vi "Lines LoadMatrixOfSessions.vi"(8 "error in (no error)":errorcluster, 9 "Input Dialog":string, 10 "Array in":string[](array[string]), 11 "Lines":string[](array[string])) -> (0 "error out":errorcluster, 2 "Array out":string[][](array[string]), 3 "Config Text List out":string[](array[string]))   [LabVIEW 2012]
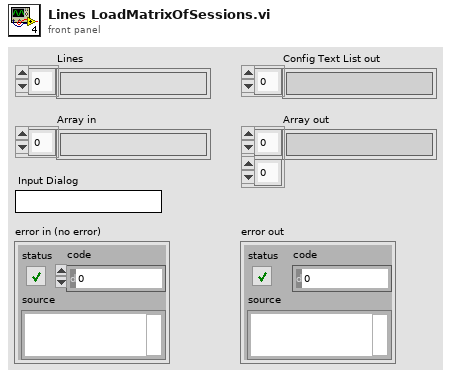
[diagram p1: front panel]
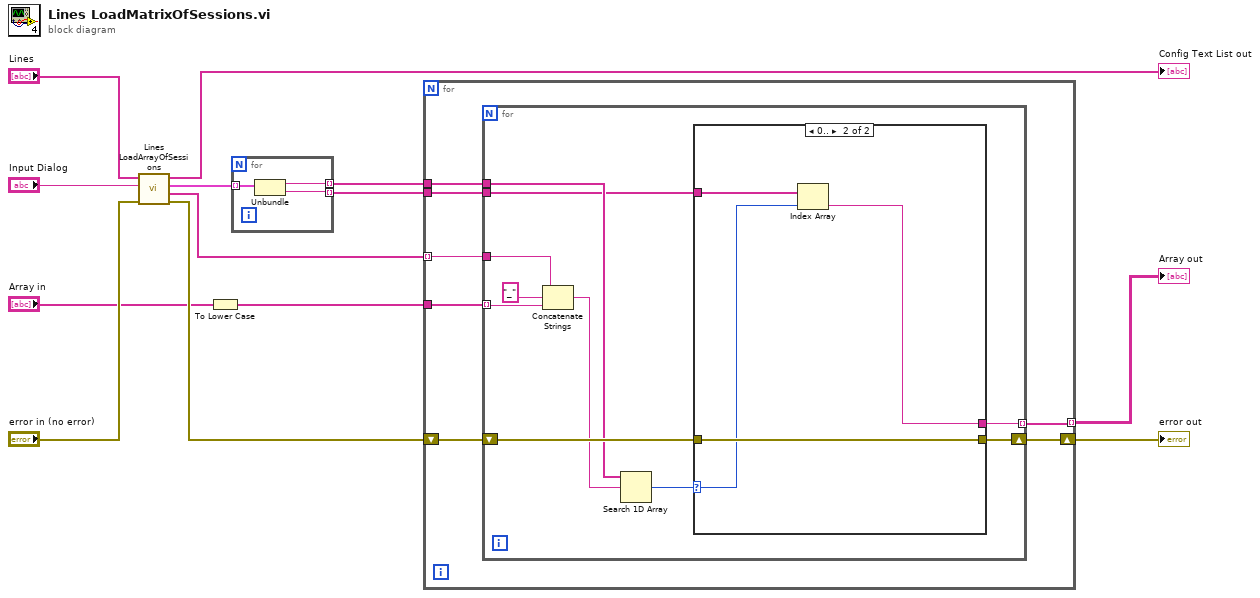
[diagram p0: block diagram]
diagram:
  n1 = call "Lines LoadArrayOfSessions.vi"("error in (no error)"="error in (no error)", "regular expression"="Input Dialog", "Lines"="Lines") -> ("error out"=w11:errorcluster, "Matched Sessions"=w6:string[], "String Config Group"=w7:cluster{"name":string, "cfg":string}[], "Config Text List out"=→"Config Text List out":string[])  [unwired: 5 in]
  n2 = To Lower Case(string="Array in") -> (all lower case string=w1:string[])
  n3 = for {
    tunnel: w7 -> [w16] mode=indexing
    tunnel: [w15] -> w8 mode=indexing
    tunnel: [w14] -> w9 mode=indexing
    n4 = Unbundle(w16) -> ("name"=w15:string, "cfg"=w14:string)
  }
  n5 = for {
    tunnel: w8 -> [w21]
    tunnel: w6 -> [w20] mode=indexing
    tunnel: w1 -> [w19]
    shift-right: [w23] -> w4
    shift-left: w11 -> [w22]
    tunnel: [w18] -> w3 mode=indexing
    tunnel: w9 -> [w17]
    n6 = for {
      shift-right: [w33] -> w23
      shift-left: w22 -> [w32]
      tunnel: w21 -> [w29]
      tunnel: w20 -> [w26]
      tunnel: [w31] -> w18 mode=indexing
      tunnel: w19 -> [w27] mode=indexing
      tunnel: w17 -> [w24]
      n7 = Concatenate Strings(w26, "_" ("string"), w27) -> (w28:string)
      n8 = Search 1D Array(1D array=w29, element=w28) -> (index of element=w25:i32)  [unwired: 1 in]
      n9 = case shown="0.." w25 {
        selector: w25 -> [_ w36]
        tunnel: [w34 w38] -> w33
        tunnel: w32 -> [w34 w38]
        tunnel: [_ w35] -> w31
        tunnel: w24 -> [_ w37]
        frame Default {
        }
        frame 0.. {
          n10 = Index Array(array=w37, index=w36) -> (element=w35:string)
        }
      }
    }
  }
  "error out" <- w4
  "Array out" <- w3
